vi "Write client proxy lookup table (clientname -_ msg queue object).vi"(8 "error in (no error)":errorcluster, 10 "client proxy lookup table (clientname -> msg queue object)":variant, 11 "Server Controller in":refnum<class "Server Controller.lvclass">) -> (0 "error out":errorcluster, 3 "Server Controller out":refnum<class "Server Controller.lvclass">)   [LabVIEW 2016, in "Server Controller.lvlib" / "Server Controller.lvclass"]
uses:
  Server Controller.lvclass
  Server Controller.lvclass/Server Controller.ctl
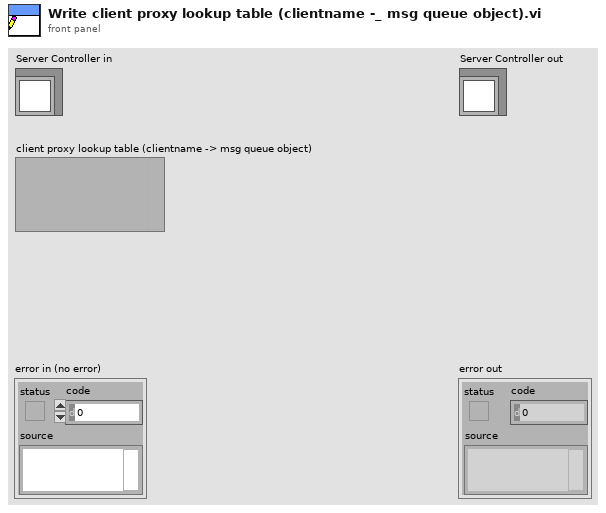
[diagram p1: front panel]
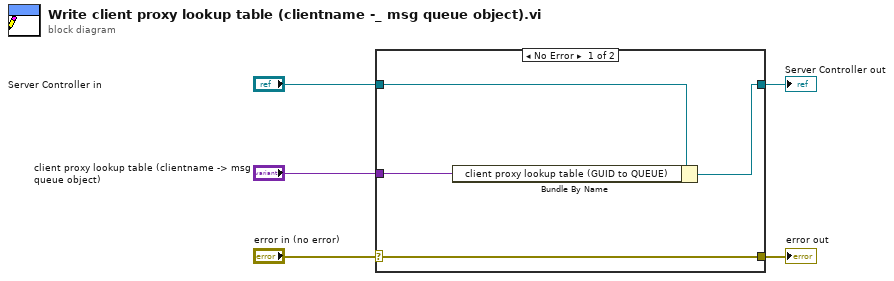
[diagram p0: block diagram]
diagram:
  n1 = case shown="No Error" "error in (no error)" {
    selector: "error in (no error)" -> [w9 w10]
    tunnel: [w9 w10] -> w4
    tunnel: [w7 w11] -> w2
    tunnel: "Server Controller in" -> [w8 w11]
    tunnel: "client proxy lookup table (clientname -> msg queue object)" -> [w6 _]
    frame No Error {
      n2 = Bundle By Name(cluster=w8, "client proxy lookup table (GUID to QUEUE)"=w6) -> (w7:refnum<class "Server Controller.lvclass">)
    }
    frame Error {
    }
  }
  "error out" <- w4
  "Server Controller out" <- w2
